vi "组件位填充与清除.vi"(8 "添/清":bool, 9 "行字母":i32=1, 10 "列数字":i32=1, 11 "PictureIN":picture) -> (3 "PictureOUT":picture)   [LabVIEW 2020]
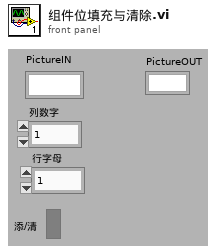
[diagram p1: front panel]
types:
  T1 = cluster{"left":i16, "top":i16, "right":i16, "bottom":i16}
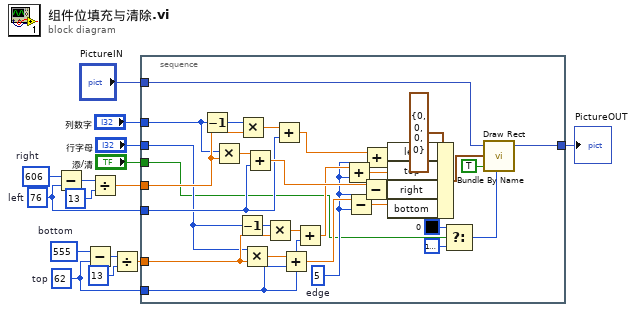
[diagram p0: block diagram]
diagram:
  w12 = i16 555  # bottom
  w4 = i16 62  # top
  w13 = i16 606  # right
  w9 = i16 76  # left
  n1 = Subtract(x=w13, y=w9) -> (x-y=w14:i16)
  n2 = Subtract(x=w12, y=w4) -> (x-y=w10:i16)
  n3 = Divide(x=w14, y=i16 13) -> (x/y=w5:dbl)
  n4 = Divide(x=w10, y=i16 13) -> (x/y=w3:dbl)
  n5 = stacked-sequence {
    tunnel: w5 -> [w24]
    tunnel: w9 -> [w23]
    tunnel: w4 -> [w22]
    tunnel: w3 -> [w21]
    tunnel: "列数字" -> [w20]
    tunnel: "行字母" -> [w19]
    tunnel: "添/清" -> [w18]
    tunnel: "PictureIN" -> [w17]
    tunnel: [w16] -> w1
    frame #0 {
      w28 = i16 5  # edge
      n6 = Decrement(x=w20) -> (x-1=w44:i32)
      n7 = Multiply(x=w20, y=w24) -> (x*y=w39:dbl)
      n8 = Decrement(x=w19) -> (x-1=w43:i32)
      n9 = Multiply(x=w44, y=w24) -> (x*y=w40:dbl)
      n10 = Multiply(x=w19, y=w21) -> (x*y=w37:dbl)
      n11 = Add(x=w39, y=w23) -> (x+y=w34:dbl)
      n12 = Multiply(x=w43, y=w21) -> (x*y=w38:dbl)
      n13 = Add(x=w40, y=w23) -> (x+y=w36:dbl)
      n14 = Add(x=w37, y=w22) -> (x+y=w30:dbl)
      n15 = Add(x=w38, y=w22) -> (x+y=w32:dbl)
      n16 = Add(x=w32, y=w28) -> (x+y=w31:dbl)
      n17 = Subtract(x=w30, y=w28) -> (x-y=w29:dbl)
      n18 = Subtract(x=w34, y=w28) -> (x-y=w33:dbl)
      n19 = Add(x=w36, y=w28) -> (x+y=w35:dbl)
      n20 = Bundle By Name(cluster=T1 {"left"=0, "top"=0, "right"=0, "bottom"=0} ("rect"), "left"=w35, "top"=w31, "right"=w33, "bottom"=w29) -> (w41:T1)
      n21 = Select(t=u32 0 ("color(black)"), s=w18, f=u32 16777226 ("color(black)")) -> (s? t:f=w27:u32)
      n22 = call <vilib>:"Draw Rect.vi"("picture"=w17, "rect"=w41, "fill?(F)"=TRUE, "color(black)"=w27) -> ("new picture"=w16:picture)  [unwired: 5 in]
    }
  }
  "PictureOUT" <- w1
